vi "串口调试助手.vi"() -> ()   [LabVIEW 2011]
uses:
  <vilib>/Instr/_visa.llb/VISA Configure Serial Port (Instr).vi
panel:
  out "十六进制整型字符串":string[](array[string])
  in  "数组 2":string[](array[string])
  out "收码区":string
  in  "单选按钮":enum32{"HEX", "字符串"}(radio)
  in  "timer":u64
  in  "连续发送":bool
  in  "时间间隔":u64
  in  "stop bits":u16(ring)=10 caption="停止位" items=["1.0"=10, "1.5"=15, "2.0"=20]
  in  "parity":u16(ring) caption="奇偶" items=["None", "Odd", "Even", "Mark", "Space"]
  in  "data bits":u16=8 caption="数据比特" min=5 max=8 step=1
  in  "baud rate":u32=9600 caption="波特率"
  in  "清除显示区":bool
  in  "停止":bool
  in  "发送":bool
  in  "串口设置":refnum<visa-resource-name>
  in  "发码区":string
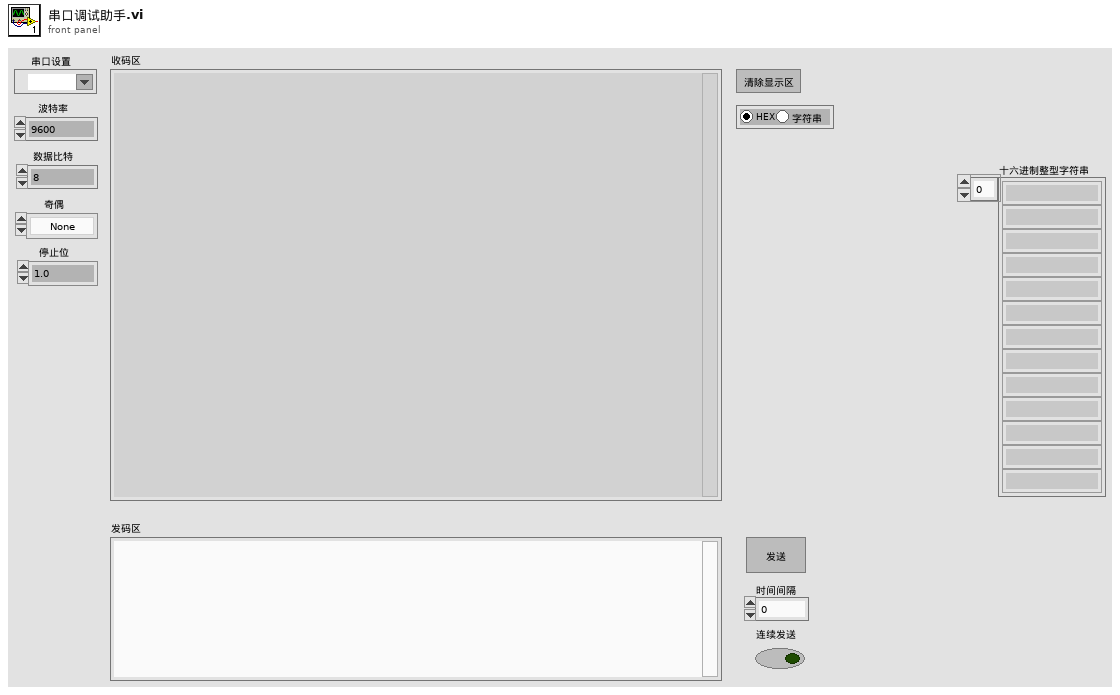
[diagram p1: front panel]
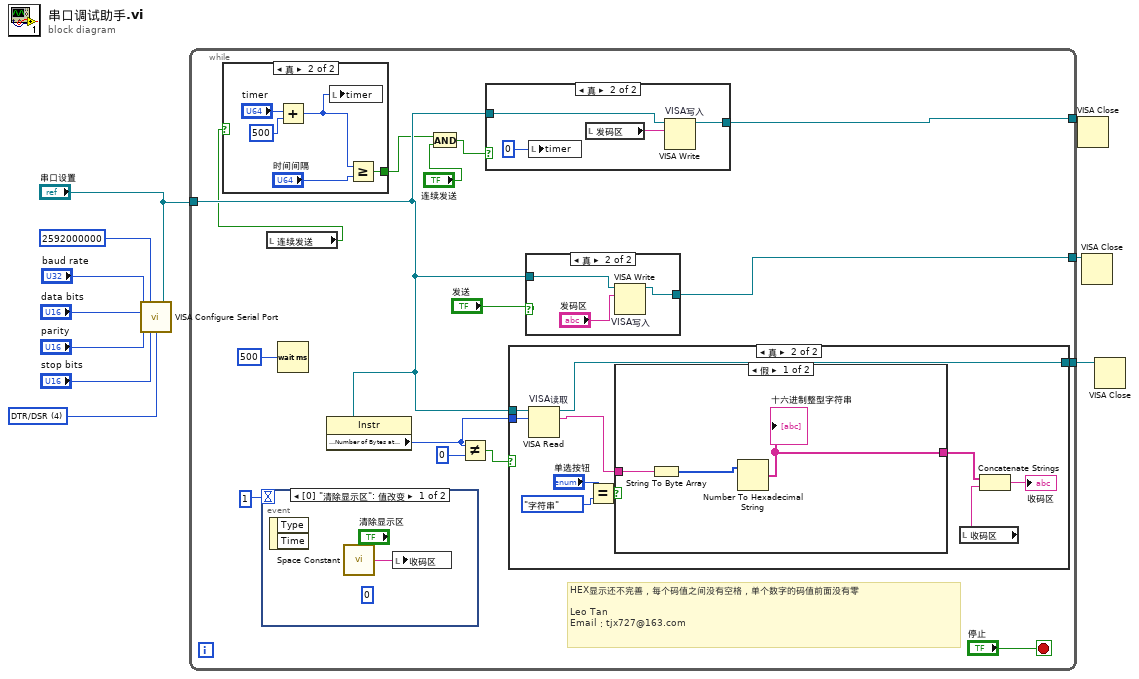
[diagram p0: block diagram]
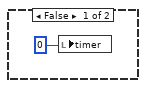
[diagram p2: hidden frame]
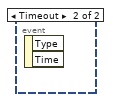
[diagram p5: hidden frame]
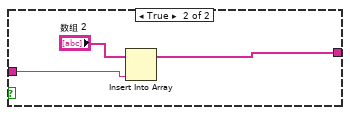
[diagram p7: hidden frame]
diagram:
  w3 = u16 4 items=["无", "XON/XOFF", "RTS/CTS", "XON/XOFF & RTS/CTS", "DTR/DSR", "XON/XOFF & DTR/DSR"] ("flow control (0:none)")
  n1 = call-poly "VISA Configure Serial Port"("VISA resource name"="串口设置", "timeout (10sec)"=u64 2592000000, "baud rate (9600)"="baud rate", "data bits (8)"="data bits", "parity (0:none)"="parity", "stop bits (10: 1 bit)"="stop bits", "flow control (0:none)"=w3) -> ()  [unwired: 7 in, 2 out]
  n2 = while {
    tunnel: "串口设置" -> [w16]
    tunnel: [w24] -> w9
    tunnel: [w18] -> w2
    tunnel: [w17] -> w1
    stop <- "停止" stop-if-true
    # "HEX显示还不完善，每个码值之间没有空格，单个数字的码值前面没有零\n\nLeo Tan\nEmail：tjx727@163.com"
    n3 = event shown="[0] \"清除显示区\": 值改变" {
      selector: _ -> [_ _]
      dyn-events: _ -> [_ _]
      timeout: 1 -> [_ _]
      event "清除显示区": Value Change {
        (unwired) 0
        n4 = event-data() -> ()  [unwired: 1 in, 2 out]
        n5 = call <vilib>:"Space Constant.vi"() -> ("String"=w39:string)
        n6 = local write "收码区"(w39) -> ()
      }
      event Timeout {
        n7 = event-data() -> ()  [unwired: 1 in, 2 out]
      }
    }
    n8 = local read "连续发送"() -> (w11:bool)
    n9 = case shown="真" w11 {
      tunnel: [_ w31] -> w12
      frame False {
        n10 = local write "timer"(0) -> ()
      }
      frame True {
        n11 = Add(x="timer", y=500) -> (x+y=w27:u64)
        n12 = local write "timer"(w27) -> ()
        n13 = Greater Or Equal?(x=w27, y="时间间隔") -> (x >= y?=w31:bool)
      }
    }
    n14 = Wait (ms)(milliseconds to wait=500) -> ()  [unwired: 1 out]
    n15 = property class="Instr"(reference=w16) -> ("Serial Settings:Number of Bytes at Serial Port"=w22:u32)  [unwired: 1 in, 2 out]
    n16 = And(x=w12, y="连续发送") -> (x .and. y?=w14:bool)
    n17 = Not Equal?(x=w22, y=u8 0) -> (x != y?=w21:bool)
    n18 = case shown="真" w14 {
      tunnel: [_ w35] -> w17
      tunnel: w16 -> [_ w34]
      frame False {
      }
      frame True {
        n19 = local write "timer"(0) -> ()
        n20 = local read "发码区"() -> (w33:string)
        n21 = VISA Write "VISA写入"(VISA resource name=w34, write buffer=w33) -> (VISA resource name out=w35:refnum<visa-resource-name>)  [unwired: 1 in, 2 out]
      }
    }
    n22 = case shown="真" w21 {
      tunnel: [_ w49] -> w24
      tunnel: w16 -> [_ w48]
      tunnel: w22 -> [_ w47]
      frame False {
      }
      frame True {
        n23 = VISA Read "VISA读取"(VISA resource name=w48, byte count=w47) -> (VISA resource name out=w49:refnum<visa-resource-name>, read buffer=w43:string)  [unwired: 1 in, 2 out]
        n24 = Equal?(x="单选按钮", y=enum32{"HEX", "字符串"}."字符串" ("单选按钮")) -> (x = y?=w44:bool)
        n25 = case shown="假" w44 {
          tunnel: w43 -> [w52 w55]
          tunnel: [w50 w54] -> w40
          frame False {
            n26 = String To Byte Array(string=w52) -> (unsigned byte array=w51:u8[])
            n27 = Number To Hexadecimal String(2:w51) -> (0:w50:string[])  [unwired: 1 in]
            "十六进制整型字符串" <- w50
          }
          frame True {
            n28 = Insert Into Array(array="数组 2", new element=w55) -> (w54:string[])  [unwired: 1 in]
          }
        }
        n29 = local read "收码区"() -> (w42:string)
        n30 = Concatenate Strings(w40, w42) -> (→"收码区":string)
      }
    }
    n31 = case shown="真" "发送" {
      tunnel: w16 -> [_ w37]
      tunnel: [_ w36] -> w18
      frame False {
      }
      frame True {
        n32 = VISA Write "VISA写入"(VISA resource name=w37, write buffer="发码区") -> (VISA resource name out=w36:refnum<visa-resource-name>)  [unwired: 1 in, 2 out]
      }
    }
  }
  n33 = VISA Close(VISA resource name=w1) -> ()  [unwired: 1 in, 1 out]
  n34 = VISA Close(VISA resource name=w2) -> ()  [unwired: 1 in, 1 out]
  n35 = VISA Close(VISA resource name=w9) -> ()  [unwired: 1 in, 1 out]
